vi "zi_OptimizeModulation.vi"(0 "zi Address":string="DEV1925", 1 "stop":bool) -> ()   [LabVIEW 2021]
doc: "Control a Zurich instrument device via the LabOne Labview API. \nRequirements: Zurich Instruments MFLI, HF2 or UHFLI \nThis example polls demod data for a given time from the instrument.\n\n© Zurich Instruments AG, www.zhinst.com"
uses:
  <vilib>/Analysis/1siggen.llb/Ramp Pattern by Samples.vi
  <instrlib>/Zurich Instruments LabOne/Public/Configure/ziSetValueDouble.vi
  <instrlib>/Zurich Instruments LabOne/Public/Configure/ziGetValueDouble.vi
  <vilib>/addons/Time Series Analysis/Statistical Analysis.llb/TSA Deviation and Variance (Array).vi
  <vilib>/addons/Time Series Analysis/Statistical Analysis.llb/TSA Mean (Array).vi
  <instrlib>/Zurich Instruments LabOne/Zurich Instruments LabOne.lvlib
  <vilib>/Analysis/NI_AALBase.lvlib
  <vilib>/addons/_Advanced Signal Processing/NI_AdvSigProcTSA.lvlib
panel:
  out "Optimal modulation voltage:":dbl
  out "Waveform Graph":dbl[](graph)=[0.007285288733195631, 0.005230055030291482, 0.006961194342232996, 0.005312173147112712]
  out "Needed chart record length:":dbl=30000.0
  out "N samples":dbl=3000.0
  in  "Sample rate":dbl=1000.0
  out "Waveform Chart":dbl[][](graph)
  in  "Update V":bool=TRUE
  out "Current V":dbl=0.34782675038719474
  in  "N voltages":dbl=10.0
  in  "Ending V":dbl=0.4
  in  "Starting V":dbl=0.2
  out "Error Out":errorcluster={"status"=TRUE, "code"=1672, "source"="Python Node in zi_OptimizeModulation.vi<APPEND>\n\nModule Path: C:\\Users\\mnopl\\Desktop\\Software\\LabVIEW\\Pseudoheterodyne\\__init__.py\nFunction Name: fit_phase_leakage"}
  in  "time":dbl=1.0 caption="recording time [s]"
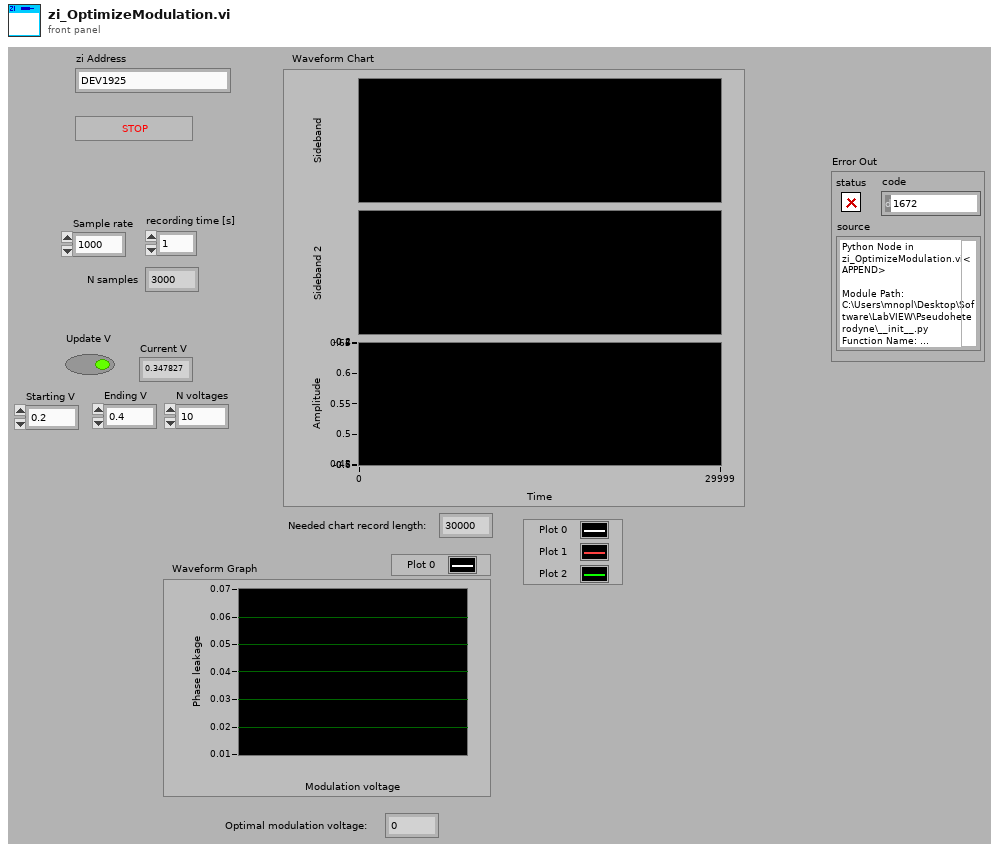
[diagram p1: front panel]
types:
  T1 = typedef "Zurich Instruments LabOne.lvlib/ziTypeHandle.ctl" = cluster{"handleValid":bool, "Conn":u64, "Path Prefix":string, "Handle":u64, "Connected":bool, "Clockbase(s)":dbl}
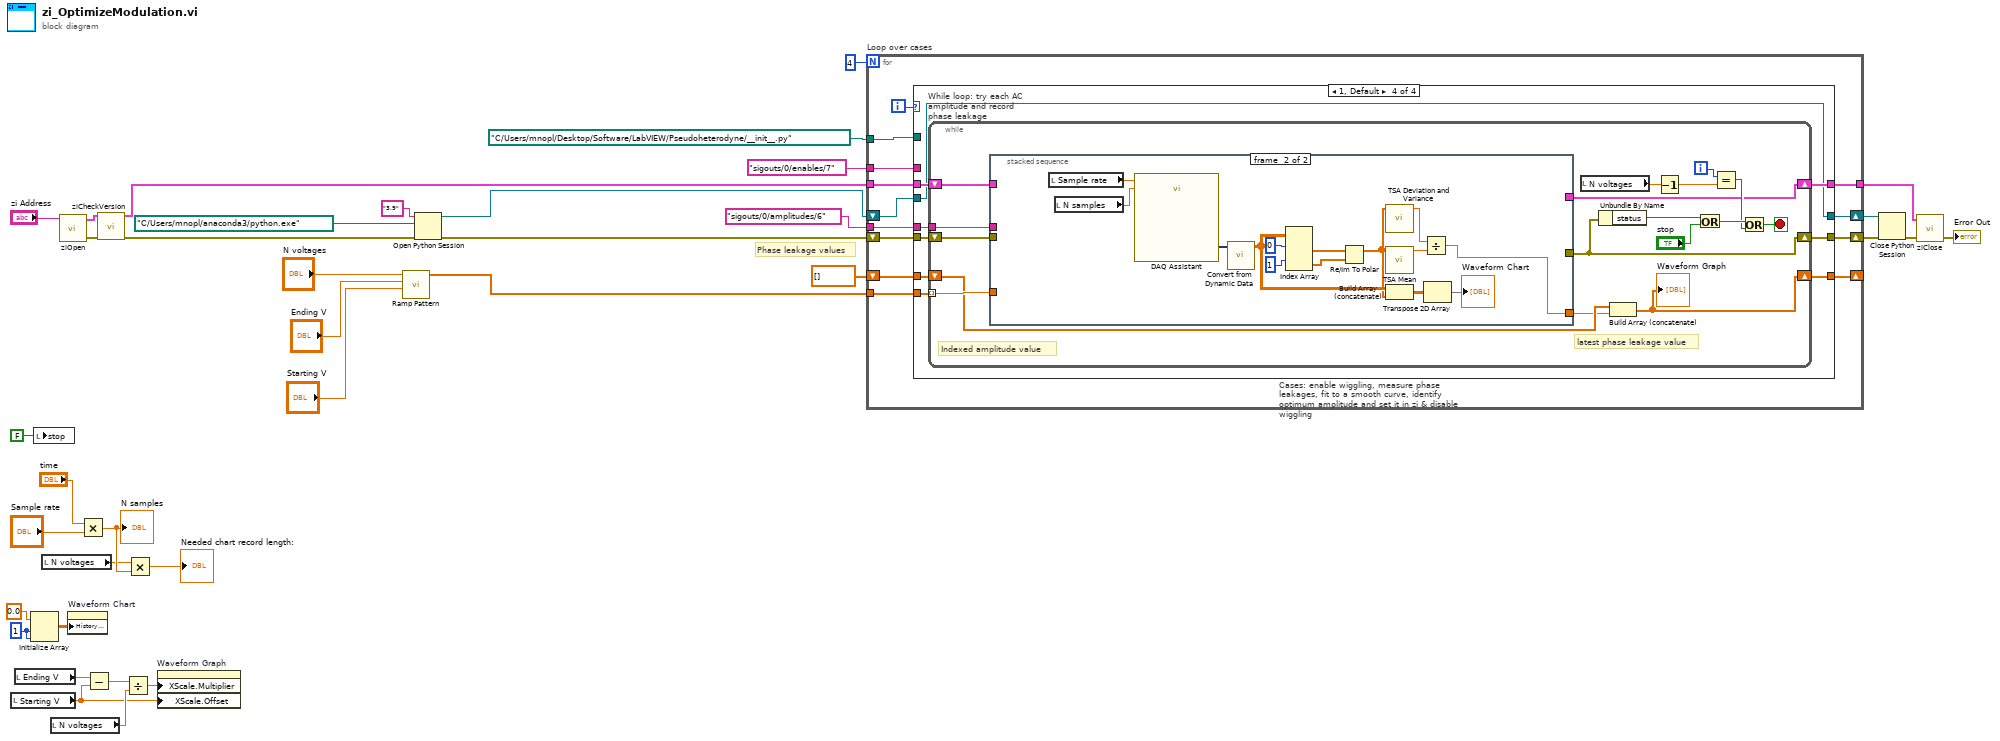
[diagram p0: block diagram]
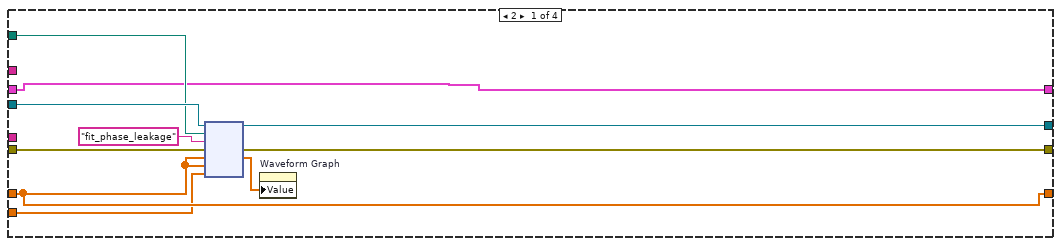
[diagram p2: hidden frame]
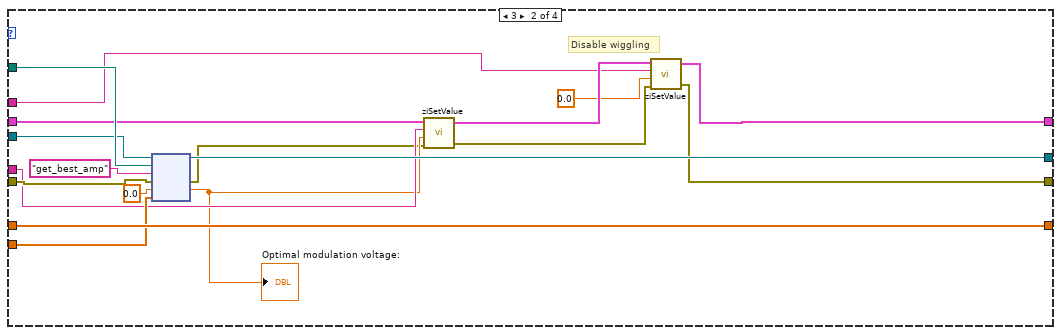
[diagram p3: hidden frame]
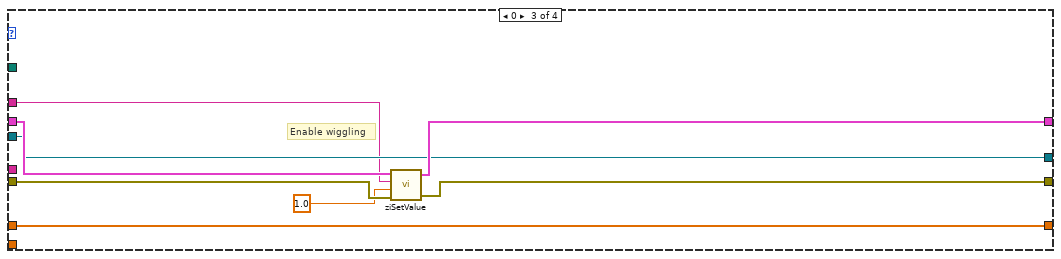
[diagram p4: hidden frame]
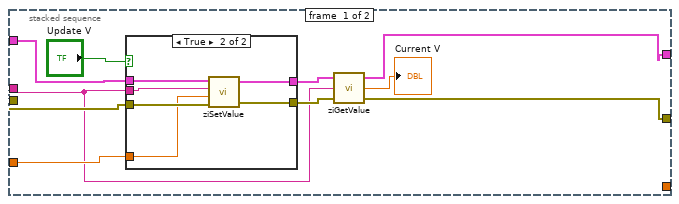
[diagram p5: hidden frame]
diagram:
  w28 = 1
  # "Phase leakage values"
  n1 = local read "Starting V"() -> (w12:dbl)
  n2 = local read "Ending V"() -> (w20:dbl)
  n3 = Initialize Array(0.0, w28, w28) -> (w21:dbl[][])
  n4 = local write "stop"(FALSE ("stop")) -> ()
  n5 = local read "N voltages"() -> (w22:dbl)
  n6 = local read "N voltages"() -> (w19:dbl)
  n7 = call <instrlib>:"ziOpen.vi"("Address"="zi Address") -> ("Error Out"=w34:errorcluster, "HandleOut"=w35:T1)  [unwired: 1 in, 3 out]
  n8 = property on="Waveform Chart" class="WFChart (strict)"("History Data"=w21) -> ()  [unwired: 2 in, 2 out]
  n9 = Multiply(x="time", y="Sample rate") -> (x*y=w23:dbl)
  "N samples" <- w23
  n10 = Subtract(x=w20, y=w12) -> (x-y=w18:dbl)
  n11 = call <instrlib>:"ziCheckVersion.vi"("Handle In"=w35, "Error In"=w34) -> ("Handle Out"=w27:T1, "Error Out"=w7:errorcluster)  [unwired: 11 in, 1 out]
  n12 = Divide(x=w18, y=w19) -> (x/y=w13:dbl)
  n13 = Multiply(x=w22, y=w23) -> (x*y=→"Needed chart record length:":dbl)
  n14 = property on="Waveform Graph" class="WFGraph (strict)"("XScale.Multiplier"=w13, "XScale.Offset"=w12) -> ()  [unwired: 2 in, 2 out]
  n15 = call-poly <vilib>:"Ramp Pattern.vi"("start"="Starting V", "end"="Ending V", "samples"="N voltages") -> ("Ramp Pattern"=w30:dbl[])  [unwired: 7 in, 1 out]
  n16 = Open Python Session(python version="3.9", python path=path "C:/Users/mnopl/anaconda3/python.exe", 3:w7) -> (session out=w5:refnum<k35>, error out=w6:errorcluster)
  n17 = for "Loop over cases" {
    N: 4 -> [_]
    tunnel: w27 -> [w49]
    shift-right: [w47] -> _
    shift-left: dbl[] [] -> [w46]
    tunnel: [w44] -> w15
    shift-right: [w45] -> w10
    shift-left: w6 -> [w43]
    tunnel: w30 -> [w50]
    shift-right: [w42] -> w11
    shift-left: w5 -> [w41]
    tunnel: path "C:/Users/mnopl/Desktop/Software/LabVIEW/Pseudoheterodyne/__init__.py" -> [w40]
    tunnel: "sigouts/0/amplitudes/6" -> [w39]
    tunnel: "sigouts/0/enables/7" -> [w38]
    i -> [w48]
    n18 = case "Cases: enable wiggling, measure phase leakages, fit to a smooth curve, identify optimum amplitude and set it in zi & disable wiggling" shown="1, Default" w48 {
      tunnel: w50 -> [w57 w71 _ w95]
      tunnel: w49 -> [w51 w70 w86 w94]
      tunnel: [w59 w73 w83 w90] -> w47
      tunnel: w46 -> [w59 w73 w83 w89]
      tunnel: [w52 w61 w81 w93] -> w45
      tunnel: [w51 w65 w85 w92] -> w44
      tunnel: w43 -> [w54 w74 w82 w91]
      tunnel: [w56 w75 w84 w88] -> w42
      tunnel: w41 -> [w55 w76 w84 w88]
      tunnel: w40 -> [w53 w77 _ _]
      tunnel: w39 -> [_ w69 _ w87]
      tunnel: w38 -> [_ w62 w80 _]
      frame 2 {
        n19 = node(w55, w53, "fit_phase_leakage", w54, w59, w59, w57) -> (w56:refnum<k35>, w52:errorcluster, w58:dbl[])  [unwired: 2 in, 2 out]
        n20 = property on="Waveform Graph" class="WFGraph (strict)"("Value"=w58) -> ()  [unwired: 2 in, 2 out]
      }
      frame 3 {
        # "Disable wiggling"
        n21 = node(w76, w77, "get_best_amp", w74, 0.0, w71) -> (w75:refnum<k35>, w67:errorcluster, w68:dbl)  [unwired: 1 in, 2 out]
        "Optimal modulation voltage:" <- w68
        n22 = call-poly <instrlib>:"ziSetValue.vi"("Error In"=w67, "Value"=w68, "Path"=w69, "Handle In"=w70) -> ("Error Out"=w64:errorcluster, "Handle Out"=w66:T1)  [unwired: 1 in]
        n23 = call-poly <instrlib>:"ziSetValue.vi"("Error In"=w64, "Value"=0.0, "Path"=w62, "Handle In"=w66) -> ("Error Out"=w61:errorcluster, "Handle Out"=w65:T1)  [unwired: 1 in]
      }
      frame 0 {
        # "Enable wiggling"
        n24 = call-poly <instrlib>:"ziSetValue.vi"("Error In"=w82, "Value"=1.0, "Path"=w80, "Handle In"=w86) -> ("Error Out"=w81:errorcluster, "Handle Out"=w85:T1)  [unwired: 1 in]
      }
      frame 1, Default {
        n25 = while "While loop: try each AC amplitude and record phase leakage" {
          shift-right: [w100] -> w92
          shift-left: w94 -> [w111]
          shift-right: [w101] -> w93
          shift-left: w91 -> [w110]
          tunnel: w95 -> [w104] mode=indexing
          shift-right: [w97] -> w90
          shift-left: w89 -> [w99]
          tunnel: w87 -> [w96]
          i -> [w105]
          stop <- w108 stop-if-true
          # "latest phase leakage value"
          # "Indexed amplitude value"
          n26 = stacked-sequence {
            tunnel: w111 -> [w122 _]
            tunnel: w110 -> [w121 _]
            tunnel: w104 -> [w120 _]
            tunnel: [w114 _] -> w101
            tunnel: [w113 _] -> w100
            tunnel: [_ w131] -> w98
            tunnel: w96 -> [w115 _]
            frame #0 {
              n27 = case shown="True" "Update V" {
                tunnel: w122 -> [w124 w130]
                tunnel: w121 -> [w123 w129]
                tunnel: w120 -> [_ w128]
                tunnel: [w124 w127] -> w118
                tunnel: [w123 w126] -> w117
                tunnel: w115 -> [_ w125]
                frame False {
                }
                frame True {
                  n28 = call-poly <instrlib>:"ziSetValue.vi"("Error In"=w129, "Value"=w128, "Path"=w125, "Handle In"=w130) -> ("Error Out"=w126:errorcluster, "Handle Out"=w127:T1)  [unwired: 1 in]
                }
              }
              n29 = call-poly <instrlib>:"ziGetValue.vi"("error in"=w117, "Path"=w115, "Handle in"=w118) -> ("error out"=w114:errorcluster, "Value"=→"Current V":dbl, "Handle out"=w113:T1)
            }
            frame #1 {
              n30 = local read "Sample rate"() -> (w135:dbl)
              n31 = local read "N samples"() -> (w136:dbl)
              n32 = call "DAQ Assistant"("rate"=w135, "number of samples"=w136) -> ("data"=w141:dynamicdata)  [unwired: 15 in, 2 out]
              n33 = call "Convert from Dynamic Data"("Dynamic Data Type"=w141) -> ("Array"=w140:dbl[][])  [unwired: 3 in]
              n34 = Index Array(array=w140, index (row) #1=0, index (row) #2=1) -> (element #1=w143:dbl[], element #2=w138:dbl[])  [unwired: 2 in]
              n35 = Re/Im To Polar(2:w138, 3:w143) -> (1:w134:dbl[])  [unwired: 1 out]
              n36 = call-poly <vilib>:"TSA Deviation and Variance.vi"("Xt"=w134) -> ("standard deviation"=w133:dbl)  [unwired: 7 in, 3 out]
              n37 = call-poly <vilib>:"TSA Mean.vi"("Xt"=w134) -> ("mean"=w132:dbl)  [unwired: 9 in, 1 out]
              n38 = Build Array (concatenate)(w140, w134) -> (w142:dbl[][])
              n39 = Divide(x=w133, y=w132) -> (x/y=w131:dbl)
              n40 = Transpose 2D Array(2D array=w142) -> (transposed array=→"Waveform Chart":dbl[][])
            }
          }
          n41 = local read "N voltages"() -> (w103:dbl)
          n42 = Unbundle By Name(w101) -> ("status"=w112:bool)
          n43 = Build Array (concatenate)(w99, w98) -> (w97:dbl[])
          "Waveform Graph" <- w97
          n44 = Decrement(x=w103) -> (x-1=w102:dbl)
          n45 = Or(x=w112, y="stop") -> (x .or. y?=w109:bool)
          n46 = Equal?(x=w105, y=w102) -> (x = y?=w106:bool)
          n47 = Or(x=w109, y=w106) -> (x .or. y?=w108:bool)
        }
      }
    }
  }
  n48 = Close Python Session(session in=w11, error in=w10) -> (11:w9:errorcluster)
  n49 = call <instrlib>:"ziClose.vi"("Error In"=w9, "Handle In"=w15) -> ("Error Out"=→"Error Out":errorcluster)  [unwired: 3 out]
